vi "PhotonPipelineResult_GetLatency_Millis.vi"(11 "PhotonPipelineResult":T1={"TargetCount"=0, "Latency_MilliSec"=0.0, "Targets"=[], "TimeStampSec"=0.0, "PhotonMultiTargetPNPResult"={"PhotonPNPResult"={"IsPresent"=FALSE, "bestReprojErr"=0.0, "altReprojErr"=0.0, "ambiguity"=0.0, "Best"={"TRANSLATION3D"={"X"=0.0, "Y"=0.0, "Z"=0.0}, "ROTATION3D"={"Q_quaternion"={"R"=1.0, "V"=[0.0, 0.0, 0.0]}}, "XF"=FALSE}, "Alt"={"TRANSLATION3D"={"X"=0.0, "Y"=0.0, "Z"=0.0}, "ROTATION3D"={"Q_quaternion"={"R"=1.0, "V"=[0.0, 0.0, 0.0]}}, "XF"=FALSE}}, "FiducialIDsUsed"=[]}} {"PhotonMultiTargetPNPResult"."PhotonPNPResult"."Alt"."TRANSLATION3D"."Z" format="%14.3f"; "PhotonMultiTargetPNPResult"."PhotonPNPResult"."Alt"."TRANSLATION3D"."Y" format="%14.3f"; "PhotonMultiTargetPNPResult"."PhotonPNPResult"."Alt"."TRANSLATION3D"."X" format="%14.3f"; "PhotonMultiTargetPNPResult"."PhotonPNPResult"."Best"."TRANSLATION3D"."Z" format="%14.3f"; "PhotonMultiTargetPNPResult"."PhotonPNPResult"."Best"."TRANSLATION3D"."Y" format="%14.3f"; "PhotonMultiTargetPNPResult"."PhotonPNPResult"."Best"."TRANSLATION3D"."X" format="%14.3f"; "Targets"."AltCameraToTarget"."TRANSLATION3D"."Z" format="%14.3f"; "Targets"."AltCameraToTarget"."TRANSLATION3D"."Y" format="%14.3f"; "Targets"."AltCameraToTarget"."TRANSLATION3D"."X" format="%14.3f"; "Targets"."BestCameraToTarget"."TRANSLATION3D"."Z" format="%14.3f"; "Targets"."BestCameraToTarget"."TRANSLATION3D"."Y" format="%14.3f"; "Targets"."BestCameraToTarget"."TRANSLATION3D"."X" format="%14.3f"}) -> (1 "TimeStampSec":dbl, 3 "Latency_MilliSec":dbl)   [LabVIEW 2019, in "PhotonVisionLib.lvlib"]
doc: "Returns the latency in the pipeline.\n\nInputs:\n - PipelineResult -- Parsed PipelineResult cluster.\n\nOutputs:\n - Latency_Millis -- The latency in the pipeline.\n - TimeStampSec -- Time stamp of packet (FPGA elapsed time) seconds"
uses:
  PhotonVisionLib.lvlib
  TypeDef/PhotonPipelineResultType.ctl
  TypeDef/PhotonTrackedTargetType.ctl
  TypeDef/TargetCornerType.ctl
  <vilib>/Rock Robotics/WPI/ThirdParty/JAS_Junk/TrajLib/TypeDef/TRANSFORM3D.ctl
  <vilib>/Rock Robotics/WPI/ThirdParty/JAS_Junk/TrajLib/TypeDef/TRANSLATION3D.ctl
  <vilib>/Rock Robotics/WPI/ThirdParty/JAS_Junk/TrajLib/TypeDef/ROTATION3D.ctl
  <vilib>/Rock Robotics/WPI/ThirdParty/JAS_Junk/TrajLib/TypeDef/QUATERNION.ctl
  TypeDef/PhotonMultiTargetPNPResultType.ctl
  TypeDef/PhotonPNPResultType.ctl
  <vilib>/Rock Robotics/WPI/ThirdParty/JAS_Junk/TrajLib/Trajectory_Library.lvlib
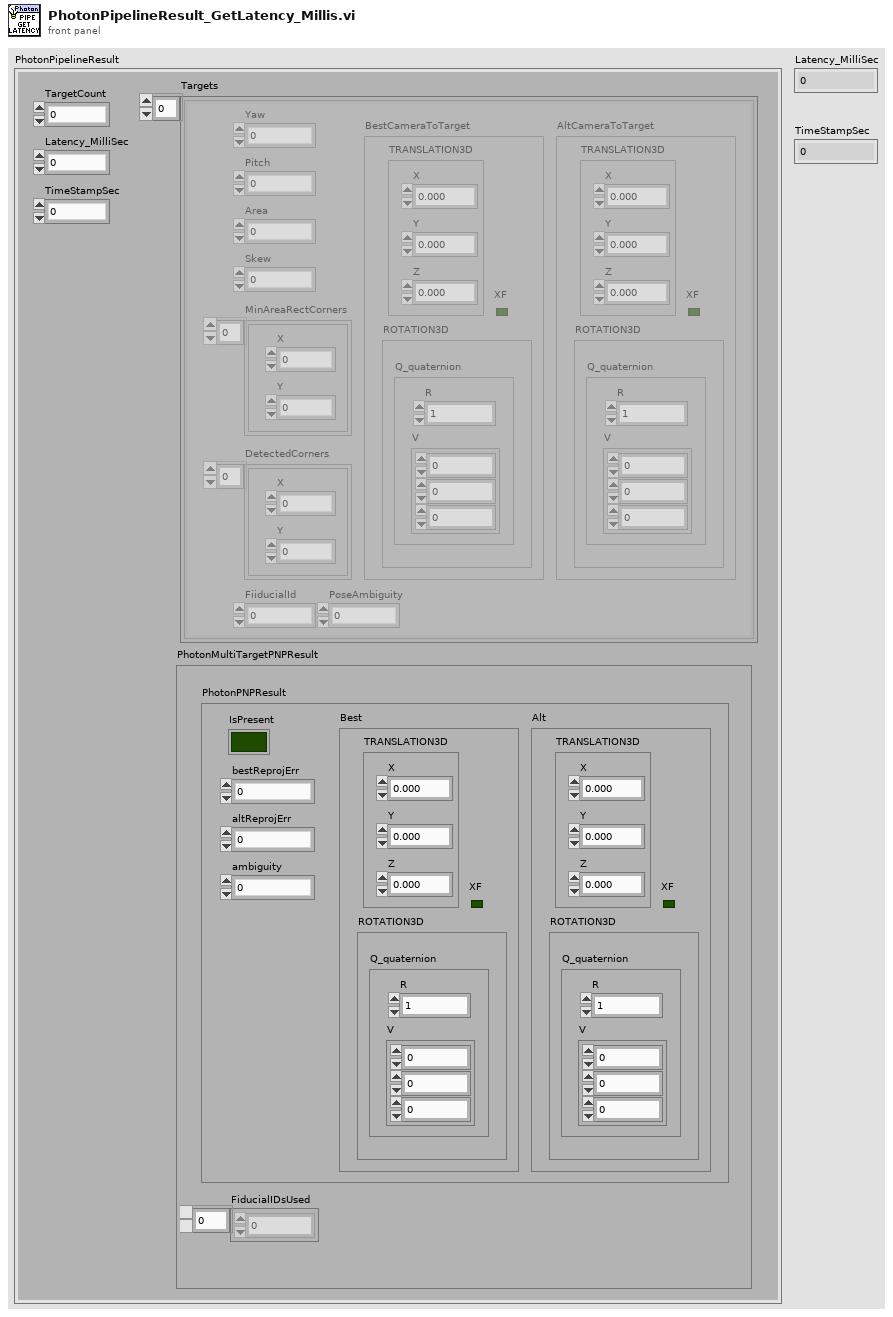
[diagram p1: front panel]
types:
  T1 = typedef "PhotonVisionLib.lvlib/PhotonPipelineResultType.ctl" = cluster{"TargetCount":i32, "Latency_MilliSec":dbl, "Targets":T2[], "TimeStampSec":dbl, "PhotonMultiTargetPNPResult":T8}
  T2 = typedef "PhotonVisionLib.lvlib/PhotonTrackedTargetType.ctl" = cluster{"Yaw":dbl, "Pitch":dbl, "Area":dbl, "Skew":dbl, "MinAreaRectCorners":T3[], "BestCameraToTarget":T4, "FiiducialId":i32, "AltCameraToTarget":T4, "PoseAmbiguity":dbl, "DetectedCorners":T3[]}
  T3 = typedef "PhotonVisionLib.lvlib/TargetCornerType.ctl" = cluster{"X":dbl, "Y":dbl}
  T4 = typedef "Trajectory_Library.lvlib/TRANSFORM3D.ctl" = cluster{"TRANSLATION3D":T5, "ROTATION3D":T6, "XF":bool}
  T5 = typedef "Trajectory_Library.lvlib/TRANSLATION3D.ctl" = cluster{"X":dbl, "Y":dbl, "Z":dbl}
  T6 = typedef "Trajectory_Library.lvlib/ROTATION3D.ctl" = cluster{"Q_quaternion":T7}
  T7 = typedef "Trajectory_Library.lvlib/QUATERNION.ctl" = cluster{"R":dbl, "V":dbl[]}
  T8 = typedef "PhotonVisionLib.lvlib/PhotonMultiTargetPNPResultType.ctl" = cluster{"PhotonPNPResult":T9, "FiducialIDsUsed":i16[]}
  T9 = typedef "PhotonVisionLib.lvlib/PhotonPNPResultType.ctl" = cluster{"IsPresent":bool, "bestReprojErr":dbl, "altReprojErr":dbl, "ambiguity":dbl, "Best":T4, "Alt":T4}
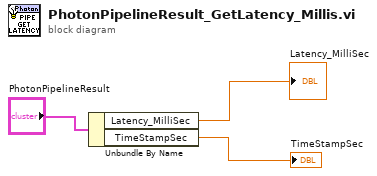
[diagram p0: block diagram]
diagram:
  n1 = Unbundle By Name("PhotonPipelineResult") -> ("Latency_MilliSec"=→"Latency_MilliSec":dbl, "TimeStampSec"=→"TimeStampSec":dbl)
